vi "APU + Event Timing 40MHz.vi"() -> ()   [LabVIEW 2013]
uses:
  IP Source/APU/Input.ctl
  IP Source/APU/Output.ctl
  IP Source/APU/Settings.ctl
  IP Source/ECU Event/Timing/Capture Output.ctl
  Event Gen Config.ctl
  IP Source/ECU Event/Timing/Measure Settings.ctl
  IP Source/Version Token.ctl
  IP Source/ECU Event/Timing/Measure Output.ctl
  IP Source/APU/Shared Settings.ctl
  <vilib>/Platform/TimedLoop/XDataNode/timing_clust.ctl
  <vilib>/Platform/TimedLoop/XDataNode/nitl_modes.ctl
  <vilib>/Platform/TimedLoop/XDataNode/wakeup.ctl
  IP Source/ECU Event/Timing/Capture Settings.ctl
  <vilib>/rvi/Emulation/niFpgaSctlEmulationGetInTimedLoop.vi
  <vilib>/rvi/Emulation/niFpgaEmulationReportErrorSimple.vi
  <vilib>/rvi/Emulation/niFpgaGetClockAttributes.vi
  <vilib>/rvi/Emulation/niFpgaCriticalErrorInLSC.vi
  IP Source/ECU Event/Timing/Measure Events (40MHz).vi
  <vilib>/Platform/TimedLoop/XDataNode/XDataNode.xnode
  <vilib>/Platform/TimedLoop/XDataNode/XDNodeRunTimeDep.lvlib
  IP Source/APU/APU.lvlib
  IP Source/ECU Event/Timing/ECU Event Timing.lvlib
  IP Source/Engine Simulation Toolkit.lvlib
panel:
  in  "go.my apu":bool
  in  "shared settings.my apu":T1 {"start" format="%#.15g"}
  out "status.spark 1":T2
  in  "est.version":T3
  in  "settings.spark 1":T4
  out "capture.spark 1.Shot 2":T5
  in  "Other Pulse Config":T6
  in  "Pulse Config":T6
  out "capture.spark 1.Shot 1":T5
  in  "settings.my apu":T7 caption="settings"
  out "output.my apu":T8 caption="output"
  in  "input.my apu":T9={"desired speed"=0.0, "reset"=TRUE} caption="input"
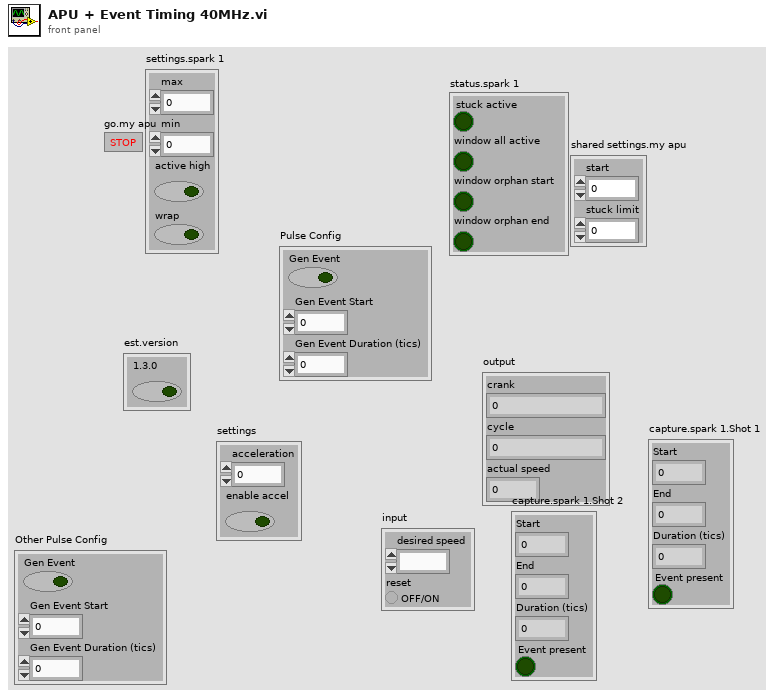
[diagram p1: front panel]
types:
  T1 = typedef "Engine Simulation Toolkit.lvlib/APU.lvlib/Shared Settings.ctl" = cluster{"start":fxp<+,17,17>, "stuck limit":fxp<+,18,18>}
  T2 = typedef "Engine Simulation Toolkit.lvlib/ECU Event Timing.lvlib/Measure Output.ctl" = cluster{"stuck active":bool, "window all active":bool, "window orphan start":bool, "window orphan end":bool}
  T3 = typedef "Engine Simulation Toolkit.lvlib/Version Token.ctl" = cluster{"1.3.0":bool}
  T4 = typedef "Engine Simulation Toolkit.lvlib/ECU Event Timing.lvlib/Measure Settings.ctl" = cluster{"max":u16, "min":u16, "active high":bool, "wrap":bool}
  T5 = typedef "Engine Simulation Toolkit.lvlib/ECU Event Timing.lvlib/Capture Output.ctl" = cluster{"Start":u16, "End":u16, "Duration (tics)":fxp<+,18,18>, "Event present":bool}
  T6 = typedef "Event Gen Config.ctl" = cluster{"Gen Event":bool, "Gen Event Start":u16, "Gen Event Duration (tics)":u32}
  T7 = typedef "Engine Simulation Toolkit.lvlib/APU.lvlib/Settings.ctl" = cluster{"acceleration":fxp<+,18,-20>, "enable accel":bool}
  T8 = typedef "Engine Simulation Toolkit.lvlib/APU.lvlib/Output.ctl" = cluster{"crank":u16, "cycle":u16, "actual speed":fxp<+/-,23,2>}
  T9 = typedef "Engine Simulation Toolkit.lvlib/APU.lvlib/Input.ctl" = cluster{"desired speed":fxp<+/-,23,2>, "reset":bool}
  T10 = typedef "XDNodeRunTimeDep.lvlib/timing_clust.ctl" = cluster{"Expected End [f-1]":u64, "Actual End [f-1]":u64, "Finished Late? [f-1]":bool, "Expected End [i-1]":u64, "Actual End [i-1]":u64, "Finished Late? [i-1]":bool, "Expected Start [i]":u64, "Actual Start [i]":u64, "Expected Start [f]":u64, "Actual Start [f]":u64, "Source Name":string, "Structure Name":string, "Period":i64, "Deadline":i64, "Offset":i64, "Start":i64, "Priority":i32, "Timeout":i32, "Mode":T11, "Wakeup Reason":T12, "Error":errorcluster, "Source Type":string, "Secondary Source Type":string, "Global End Time":u64, "Global Start Time":u64, "Frame Duration":u64, "Iteration Duration":u64, "Assigned CPU":i32, "I/O Scan Engine Mode":u32}
  T11 = typedef "XDNodeRunTimeDep.lvlib/nitl_modes.ctl" = enum32{"No Change", "Process missed periods, maintain original phase", "Discard missed periods, maintain original phase", "Process missed periods, ignore original phase", "Discard missed periods, ignore original phase"}
  T12 = typedef "XDNodeRunTimeDep.lvlib/wakeup.ctl" = enum32{"Normal", "Aborted", "Asynchronous wakeup", "Timing source error", "Timed loop error", "Timeout"}
  T13 = typedef "Engine Simulation Toolkit.lvlib/APU.lvlib/Register Bus.ctl" = cluster{"Speed":refnum<k21>, "Crank Angle":refnum<k21>, "Cycle Angle":refnum<k21>, "Crank Count":refnum<k21>, "Cycle Count":refnum<k21>, "1.25 MHz Counter":refnum<k21>, "Crank Rollover":refnum<k21>, "Cycle Rollover":refnum<k21>, "shared settings":T1}
  T14 = typedef "Engine Simulation Toolkit.lvlib/ECU Event Timing.lvlib/Capture Settings.ctl" = u8
  T15 = typedef "Engine Simulation Toolkit.lvlib/ECU Event Timing.lvlib/Measured Data.ctl" = cluster{"start":u16, "end":u16, "duration (tics)":fxp<+,18,18>, "window end":bool, "window begin":bool, "pulse end":bool, "pulse #":u8}
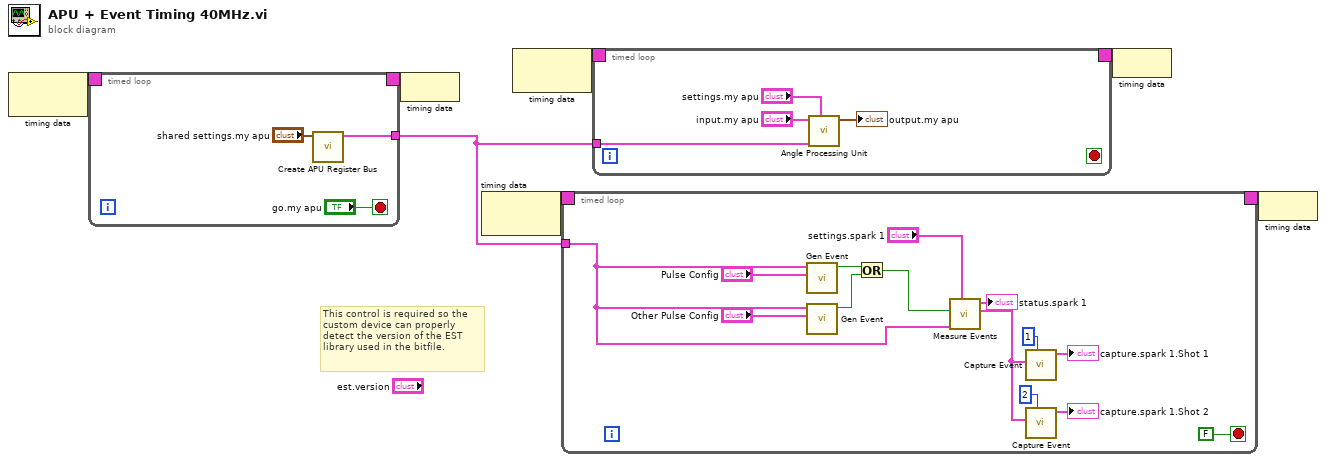
[diagram p0: block diagram]
diagram:
  # "This control is required so the custom device can properly detect the version of the EST library used in the bitfile."
  n1 = node-c288() -> (w4:T10)  [unwired: 1 in]
  n2 = timed-loop {
    timing: w4 -> [_]
    timing-out: [_] -> w3
    tunnel: [w10] -> w5
    stop <- "go.my apu" stop-if-true
    n3 = call "Create APU Register Bus.vi"("shared settings.<user name>"="shared settings.my apu") -> ("register bus"=w10:T13)  [unwired: 10 in]
  }
  n4 = node-c288(w3) -> ()
  n5 = node-c288() -> (w2:T10)  [unwired: 1 in]
  n6 = node-c288() -> (w7:T10)  [unwired: 1 in]
  n7 = timed-loop {
    tunnel: w5 -> [w20]
    timing: w2 -> [_]
    timing-out: [_] -> w1
    stop <- FALSE stop-if-true
    n8 = call "Gen Event.vi"("Event Config"="Pulse Config", "register bus"=w20) -> ("Event"=w25:bool)  [unwired: 9 in]
    n9 = call "Gen Event.vi"("Event Config"="Other Pulse Config", "register bus"=w20) -> ("Event"=w22:bool)  [unwired: 9 in]
    n10 = Or(x=w25, y=w22) -> (x .or. y?=w19:bool)
    n11 = call-poly "Measure Events.vi"("settings.<user name>"="settings.spark 1", "register bus"=w20, "event"=w19) -> ("measured data"=w17:T15, "status.<user name>"=→"status.spark 1":T2)  [unwired: 7 in]
    n12 = call "Capture Event.vi"("event # to capture"=T14 1 ("Settings.my event"), "measured data"=w17) -> ("capture.<user name>"=→"capture.spark 1.Shot 1":T5)  [unwired: 9 in]
    n13 = call "Capture Event.vi"("event # to capture"=T14 2 ("Settings.my other event"), "measured data"=w17) -> ("capture.<user name>"=→"capture.spark 1.Shot 2":T5)  [unwired: 9 in]
  }
  n14 = timed-loop {
    timing: w7 -> [_]
    timing-out: [_] -> w6
    tunnel: w5 -> [w29]
    stop <- _ stop-if-true
    n15 = call "Angle Processing Unit.vi"("settings.<user name>"="settings.my apu", "register bus"=w29, "input.<user name>"="input.my apu") -> ("output.<user name>"=→"output.my apu":T8)  [unwired: 8 in]
  }
  n16 = node-c288(w6) -> ()
  n17 = node-c288(w1) -> ()
